vi "Stop ILC.vi"(8 "error in (no error)":errorcluster, 11 "Model in":refnum<class "Model.lvclass">) -> (0 "error out":errorcluster, 3 "Model out":refnum<class "Model.lvclass">)   [LabVIEW 2016, in "Model.lvclass"]
uses:
  Model.lvclass
  Model.lvclass/Model.ctl
  Modbus/DesktopModbus/DesktopModbus.lvclass
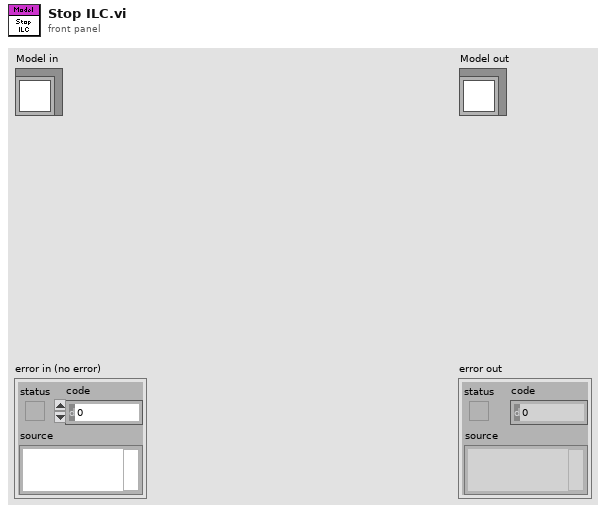
[diagram p1: front panel]
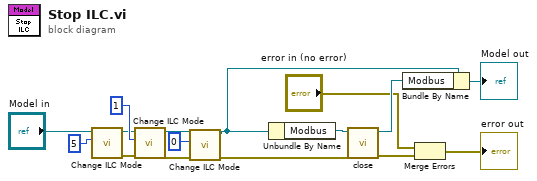
[diagram p0: block diagram]
diagram:
  n1 = call "Change ILC Mode.vi"("Mode"=u16 5, "Model in"="Model in") -> ("error out"=w16:errorcluster, "Model out"=w14:refnum<class "Model.lvclass">)  [unwired: 8 in]
  n2 = call "Change ILC Mode.vi"("error in (no error)"=w16, "Mode"=u16 1, "Model in"=w14) -> ("error out"=w4:errorcluster, "Model out"=w5:refnum<class "Model.lvclass">)  [unwired: 7 in]
  n3 = call "Change ILC Mode.vi"("error in (no error)"=w4, "Mode"=u16 0, "Model in"=w5) -> ("error out"=w1:errorcluster, "Model out"=w2:refnum<class "Model.lvclass">)  [unwired: 7 in]
  n4 = Unbundle By Name(w2) -> ("Modbus"=w10:refnum<class "DesktopModbus.lvclass">)
  n5 = call "close.vi"("error in (no error)"=w1, "DesktopModbus in"=w10) -> ("error out"=w12:errorcluster, "DesktopModbus out"=w11:refnum<class "DesktopModbus.lvclass">)  [unwired: 8 in]
  n6 = Bundle By Name(cluster=w2, "Modbus"=w11) -> (→"Model out":refnum<class "Model.lvclass">)
  n7 = Merge Errors("error in (no error)", w12) -> (→"error out":errorcluster)
